vi "SmartBathroom.vi"() -> ()   [LabVIEW 2020]
uses:
  <vilib>/Instr/_visa.llb/VISA Configure Serial Port (Instr).vi
panel:
  out "?":bool
  out "Muc nuoc":dbl(slide) scale=0.0..100.0
  out "?":bool
  out "?":bool
  out "Nhiet do\nDo am\nDo am":dbl(slide) scale=0.0..100.0
  out "Do am":dbl(slide) scale=0.0..100.0
  in  "stop":bool
  in  "VISA resource name":refnum<visa-resource-name>
  # "INDICATORS"
  # "Alarm"
  # "Nhiet do"
  # "Do am"
  # "Muc nuoc"
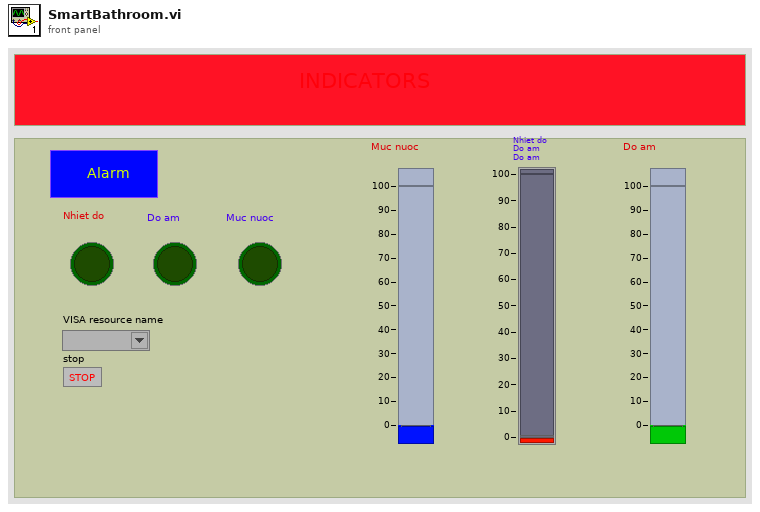
[diagram p1: front panel]
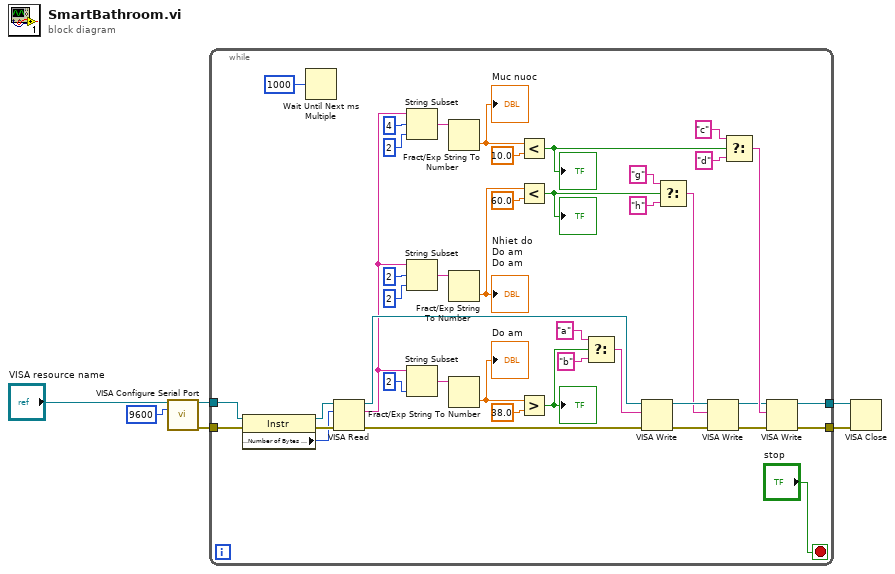
[diagram p0: block diagram]
diagram:
  n1 = call-poly "VISA Configure Serial Port"("VISA resource name"="VISA resource name", "baud rate (9600)"=u32 9600) -> ("VISA resource name out"=w6:refnum<visa-resource-name>, "error out"=w3:errorcluster)  [unwired: 12 in]
  n2 = while {
    tunnel: w6 -> [w17]
    tunnel: [w13] -> w5
    tunnel: [w12] -> w4
    tunnel: w3 -> [w16]
    stop <- "stop" stop-if-true
    n3 = property class="Instr"(reference=w17, error in=w16) -> (reference out=w48:refnum<visa-resource-name>, error out=w47:errorcluster, "Serial Settings:Number of Bytes at Serial Port"=w46:u32)
    n4 = Wait Until Next ms Multiple(millisecond multiple=u32 1000 ("milliseconds to wait")) -> ()  [unwired: 1 out]
    n5 = VISA Read(VISA resource name=w48, byte count=w46, error in (no error)=w47) -> (VISA resource name out=w11:refnum<visa-resource-name>, read buffer=w10:string, error out=w39:errorcluster)  [unwired: 1 out]
    n6 = String Subset(string=w10, offset (0)=4, length (rest)=2 ("length (rest)")) -> (substring=w23:string)
    n7 = String Subset(string=w10, offset (0)=2, length (rest)=2 ("length (rest)")) -> (substring=w40:string)
    n8 = String Subset(string=w10, length (rest)=2 ("length (rest)")) -> (substring=w41:string)  [unwired: 1 in]
    n9 = Fract/Exp String To Number(string=w23) -> (number=w22:dbl)  [unwired: 3 in, 1 out]
    "Muc nuoc" <- w22
    n10 = Fract/Exp String To Number(string=w40) -> (number=w28:dbl)  [unwired: 3 in, 1 out]
    "Nhiet do\nDo am\nDo am" <- w28
    n11 = Fract/Exp String To Number(string=w41) -> (number=w38:dbl)  [unwired: 3 in, 1 out]
    "Do am" <- w38
    n12 = Less?(x=w22, y=10.0) -> (x < y?=w7:bool)
    "?" <- w7
    n13 = Less?(x=w28, y=60.0) -> (x < y?=w25:bool)
    "?" <- w25
    n14 = Greater?(x=w38, y=38.0) -> (0:w26:bool)
    "?" <- w26
    n15 = Select(t="a", s=w26, f="b") -> (s? t:f=w36:string)
    n16 = VISA Write(VISA resource name=w11, write buffer=w36, error in (no error)=w39) -> (VISA resource name out=w32:refnum<visa-resource-name>, error out=w33:errorcluster)  [unwired: 1 out]
    n17 = Select(t="g", s=w25, f="h") -> (s? t:f=w27:string)
    n18 = VISA Write(VISA resource name=w32, write buffer=w27, error in (no error)=w33) -> (VISA resource name out=w15:refnum<visa-resource-name>, error out=w14:errorcluster)  [unwired: 1 out]
    n19 = Select(t="c", s=w7, f="d") -> (s? t:f=w18:string)
    n20 = VISA Write(VISA resource name=w15, write buffer=w18, error in (no error)=w14) -> (VISA resource name out=w13:refnum<visa-resource-name>, error out=w12:errorcluster)  [unwired: 1 out]
  }
  n21 = VISA Close(VISA resource name=w5, error in (no error)=w4) -> ()  [unwired: 1 out]
